vi "MDriveErrorCodes.vi"(4 "Error Code":string) -> (1 "Error Description":string)   [LabVIEW 2010]
panel:
  in  "MDrive Error Strings":string="Programming Reference \nError Code Fault \n0 No Error \nI/O Errors \nError Code 6 An I/O is already set to this type. Applies to non-General Purpose I/O.    \nError Code 8 Tried to set an I/O to an incorrect I/O type. \nError Code 9 Tried to write to I/O set as Input or is ÒTYPEDÓ. \nError Code 10 Illegal I/O number. \nError Code 11 Incorrect CLOCK type. \nError Code 12 Illegal Trip / Capture \nData Errors \nError Code 20 Tried to set unknown variable or flag. Trying to set an undefined variable of flag.  Also could be a typo. \nError Code 21 Tried to set an incorrect value. Many variables have a range such as the Run Current (RC) which is 1 to 100%. As an example, you cannot set the RC to 110%. \nError Code 22 VI is set greater than or equal to VM. The Initial Velocity is set equal to, or higher than the Maximum Velocity. VI must be less than VM. \nError Code 23 VM is set less than or equal to VI. The Maximum Velocity is set equal to, or lower than the Initial Velocity. VM must be greater than VI. \nError Code 24 Illegal data entered. Data has been entered that the device does not understand. \nError Code 25 Variable or flag is read only. Read only flags and variables cannot be set. \nError Code 26 Variable or flag is not allowed to be incremented or decremented. IC and DC cannot be used on variables or flags such as Baud and Version. \nError Code 27 Trip not defined.Trying to enable a trip that has not yet been defined. \nError Code 28 WARNING! Trying to redefine a program label or variable. This can be caused when you download a program over a program already saved. Before downloading a new or edited program, type <FD> and press ENTER to return the device to the Factory \nDefaults. You may also type <CP> and press ENTER to Clear the Program. \nError Code 29 Trying to redefine a built in command, variable or flag. \nError Code 30 Unknown label or user variable. Trying to Call or Branch to a Label or Variable that has not yet been defined. \nError Code 31 Program label or user variable table is full. The table has a maximum capacity of 22 labels and/or user variables. \nError Code 32 Trying to set a label (LB). You cannot name a label and then try to set it to a value. Example: Lable P1 (LB P1 ). The P1 cannot be used to set a variable such as P1=1000. \nError Code 33 Trying to SET an Instruction. \nError Code 34 Trying to Execute a Variable or Flag \nError Code 35 Trying to Print Illegal Variable or Flag \nError Code 36 Illegal Motor Count to Encoder Count Ratio \nError Code 37 Command, Variable or Flag Not Available in Drive \nError Code 38 Missing parameter separator \nError Code 39 Trip on Position and Trip on Relative Distance not allowed together\nProgram Errors \nError Code 40 Program not running. If HOLD (H) is entered in Immediate Mode and a program is not running. \nError Code 41 Not Used. \nError Code 42 Illegal program address. Tried to Clear, List, Execute, etc. an incorrect Program address. \nError Code 43 Tried to overflow program stack. Calling a Sub-Routine or Trip Routine with no Return. \nError Code 44 Program locked. User Programs can be Locked with the <LK> command. Once Locked, the program cannot be listed or edited in any way. \nError Code 45 Trying to Overflow Program Space. \nError Code 46 Not in Program Mode. \nError Code 47 Tried to Write to Illegal Flash Address \nError Code 48 Program Execution stopped by I/O set as Stop. \nCommunications Errors \nError Code 60 Not used \nError Code 61 Trying to set illegal BAUD rate. The only Baud Rates accepted are those listed on the Properties Page of IMS Terminal. (4,800, 9,600, 19,200, 38,400, 115,200) \nError Code 62 IV already pending or IF Flag already TRUE. \nSystem Errors \nError Code 70 FLASH Check Sum Fault \nError Code 71 Internal Temperature Warning, 10C to Shutdown \nError Code 72 Internal Over TEMP Fault, Disabling Drive \nError Code 73 Tried to SAVE while moving \nError Code 74 Tried to Initialize Parameters (IP) or Clear Program (CP) while Moving \nError Code 75 Linear Overtemperature Error (For units without Internal Over Temp) \nMotion Errors \nError Code 80 HOME switch not defined. Attempting to do a HOME (H) sequence but the Home Switch has not yet been defined. \nError Code 81 HOME type not defined. The HOME (HM or HI) Command has been programmed but with no type or an illegal type. (Types = 1, 2, 3, or 4) \nError Code 82 Went to both LIMITS and did not find home. The motion encroached both limits but did not trip the Home switch. Indicates a possible bad switch or a bad circuit. \nError Code 83 The LIMIT switch in the plus direction was tripped. \nError Code 84 The LIMIT switch in the minus direction was tripped. \nError Code 85 MA or MR isnÕt allowed during a HOME and a HOME isnÕt allowed while the device is in motion. \nError Code 86 Stall detected. The Stall Flag (ST) has been set to 1. \nError Code 87 In Clock Mode, JOG not allowed \nError Code 88 Following Error \nError Code 89 Reserved \nError Code 90 Motion Variables are too low switching to EE=1 \nError Code 91 Motion stopped by I/O set as Stop. \nError Code 92 Position Error in Closed loop. motor will attempt to position the shaft within the deadband, After failing 3 attempts Error 92 will be generated. Axis will continue to function normally. \nError Code 93 MR or MA not allowed while correcting position at end of previous MR or MA."
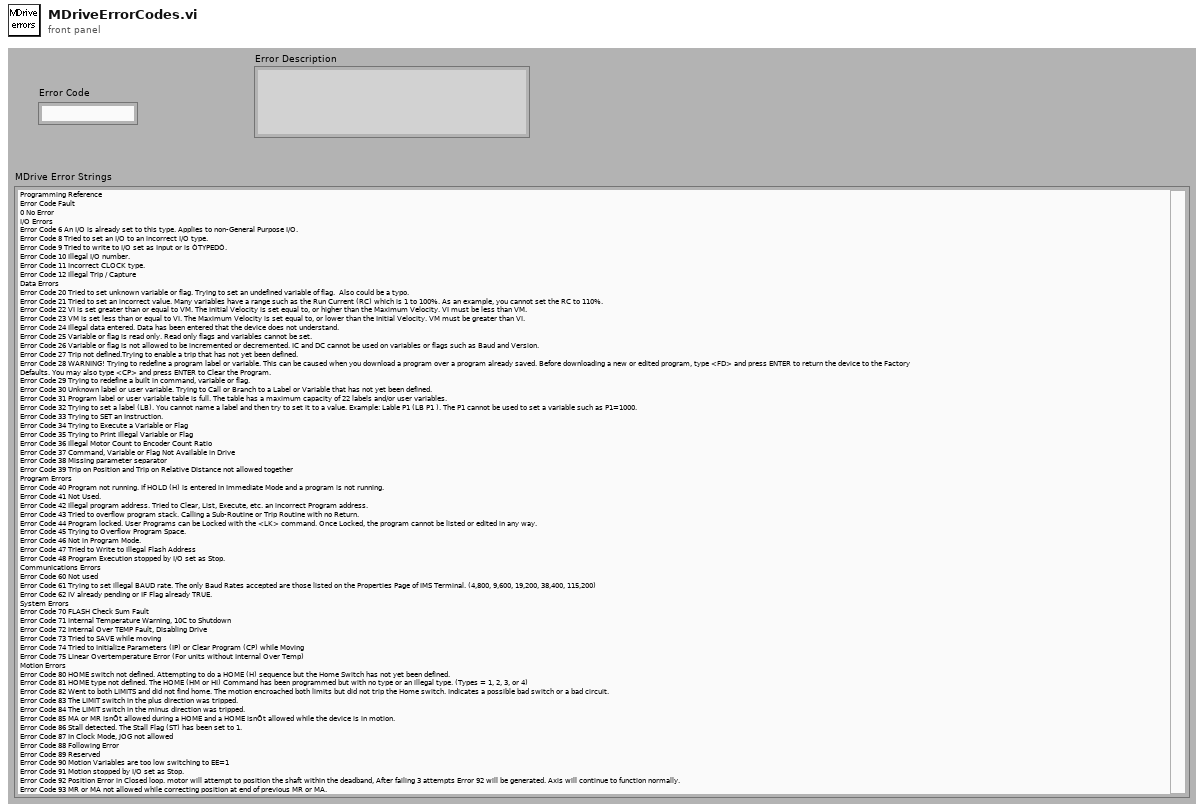
[diagram p1: front panel]
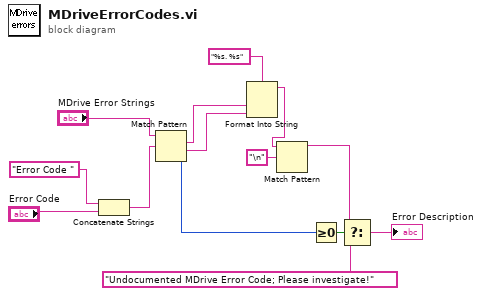
[diagram p0: block diagram]
diagram:
  n1 = Concatenate Strings("Error Code ", "Error Code") -> (w5:string)
  n2 = Match Pattern(string="MDrive Error Strings", regular expression=w5) -> (match substring=w4:string, after substring=w3:string, offset past match=w12:i32)  [unwired: 2 out]
  n3 = Format Into String(format string="%s. %s", w4, w3) -> (resulting string=w1:string)  [unwired: 2 in, 1 out]
  n4 = Match Pattern(string=w1, regular expression="\n") -> (before substring=w10:string)  [unwired: 4 out]
  n5 = Greater Or Equal To 0?(x=w12) -> (x >= 0?=w11:bool)
  n6 = Select(t=w10, s=w11, f="Undocumented MDrive Error Code; Please investigate!") -> (s? t:f=→"Error Description":string)
